vi "Prueffer Code Generator.vi"(11 "Array":i32[](array[numeric])) -> (3 "Adjacency Matrix":T1)   [LabVIEW 2016]
uses:
  <vilib>/Analysis/Matrix/Datatypes/RealMatrix.ctl
  <vilib>/Analysis/Matrix/NI_Matrix.lvlib
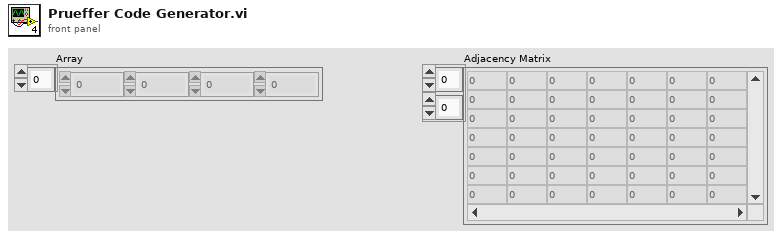
[diagram p1: front panel]
types:
  T1 = typedef "NI_Matrix.lvlib/RealMatrix.ctl" = dbl[][]
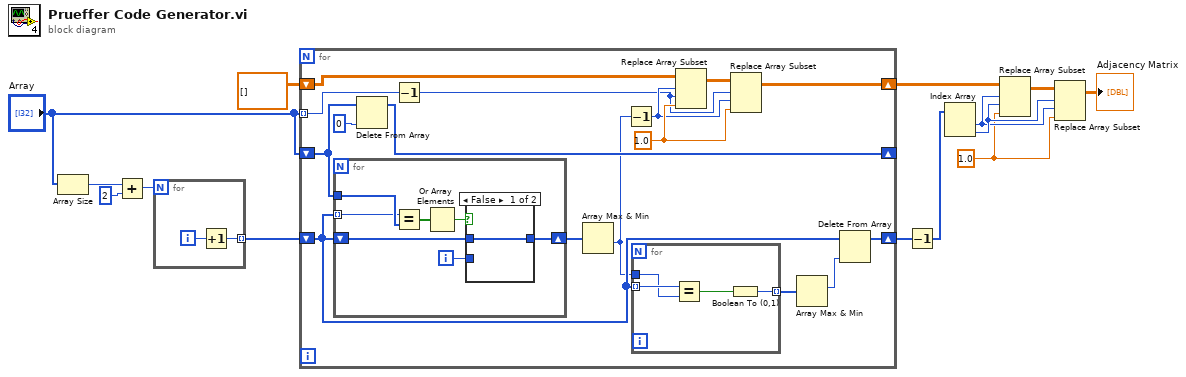
[diagram p0: block diagram]
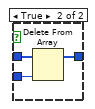
[diagram p2: hidden frame]
diagram:
  w3 = 1.0 ("new element/submatrix")
  n1 = Array Size(array="Array") -> (size(s)=w14:i32)
  n2 = Add(x=w14, y=2) -> (x+y=w13:i32)
  n3 = for {
    N: w13 -> [_]
    tunnel: [w15] -> w11 mode=indexing
    i -> [w16]
    n4 = Increment(x=w16) -> (x+1=w15:i32)
  }
  n5 = for {
    shift-right: [w25] -> w7
    shift-left: w11 -> [w20]
    tunnel: "Array" -> [w27] mode=indexing
    shift-right: [w30] -> w2
    shift-left: T1 [] ("matrix") -> [w24]
    shift-right: [w21] -> _
    shift-left: "Array" -> [w23]
    w31 = 1.0 ("new element/submatrix")
    n6 = for {
      tunnel: w20 -> [w41] mode=indexing
      tunnel: w23 -> [w43]
      shift-right: [w37] -> w26
      shift-left: w20 -> [w39]
      i -> [w38]
      n7 = Equal?(x=w41, y=w43) -> (x = y?=w42:bool[])
      n8 = Or Array Elements(Boolean array=w42) -> (logical OR=w40:bool)
      n9 = case shown="False" w40 {
        tunnel: w39 -> [w44 w47]
        tunnel: w38 -> [_ w46]
        tunnel: [w44 w45] -> w37
        frame False {
        }
        frame True {
          n10 = Delete From Array(array=w47, index=w46) -> (array with subset deleted=w45:i32[])  [unwired: 1 in, 1 out]
        }
      }
    }
    n11 = Delete From Array(array=w23, index=0) -> (array with subset deleted=w21:i32[])  [unwired: 1 in, 1 out]
    n12 = Decrement(x=w27) -> (x-1=w28:i32)
    n13 = Array Max & Min(array=w26) -> (min value=w19:i32)  [unwired: 3 out]
    n14 = Decrement(x=w19) -> (x-1=w29:i32)
    n15 = for {
      tunnel: w20 -> [w36] mode=indexing
      tunnel: w19 -> [w35]
      tunnel: [w33] -> w18 mode=indexing
      n16 = Equal?(x=w36, y=w35) -> (x = y?=w34:bool)
      n17 = Boolean To (0,1)(Boolean=w34) -> (0, 1=w33:i16)
    }
    n18 = Replace Array Subset(array=w24, new element=w31, index (row)=w29, index (col)=w28) -> (w32:T1)
    n19 = Replace Array Subset(array=w32, new element=w31, index (row)=w28, index (col)=w29) -> (w30:T1)
    n20 = Array Max & Min(array=w18) -> (max index (indices)=w17:i32)  [unwired: 3 out]
    n21 = Delete From Array(array=w20, index=w17) -> (array with subset deleted=w25:i32[])  [unwired: 1 in, 1 out]
  }
  n22 = Decrement(x=w7) -> (x-1=w6:i32[])
  n23 = Index Array(array=w6) -> (element #1=w4:i32, element #2=w5:i32)  [unwired: 2 in]
  n24 = Replace Array Subset(array=w2, new element=w3, index (row)=w4, index (col)=w5) -> (w8:T1)
  n25 = Replace Array Subset(array=w8, new element=w3, index (row)=w5, index (col)=w4) -> (→"Adjacency Matrix":T1)
